vi "setMoveMode.vi"(0 "Controller in":refnum<class "_Controller.lvclass">, 2 "mode":T1, 5 "error in (no error)":errorcluster) -> (14 "Controller out":refnum<class "_Controller.lvclass">, 17 "success?":bool, 18 "response":string, 19 "error out":errorcluster)   [LabVIEW 2020, in "classes.lvlib" / "_Controller.lvclass"]
doc: "Sets the Move Mode to either ABSOLUTE or INCREMENTAL\n\nProduced By:\n\n<B>Kod Integrations, LLC</B>\n4835 Marianne Drive\nMount Airy, MD 21771\nhttp://www.kodintegrations.com\nemail: info@kodintegrations.com\nphone: (240) 687-1288"
uses:
  _Controller.lvclass
  common/controls/move_mode.ctl
  libraries/common.lvlib
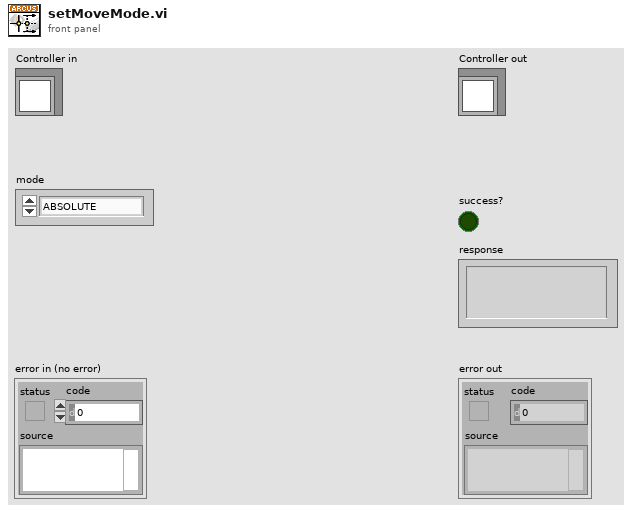
[diagram p1: front panel]
types:
  T1 = typedef "common.lvlib/move_mode.ctl" = enum16{"ABSOLUTE", "INCREMENTAL"}
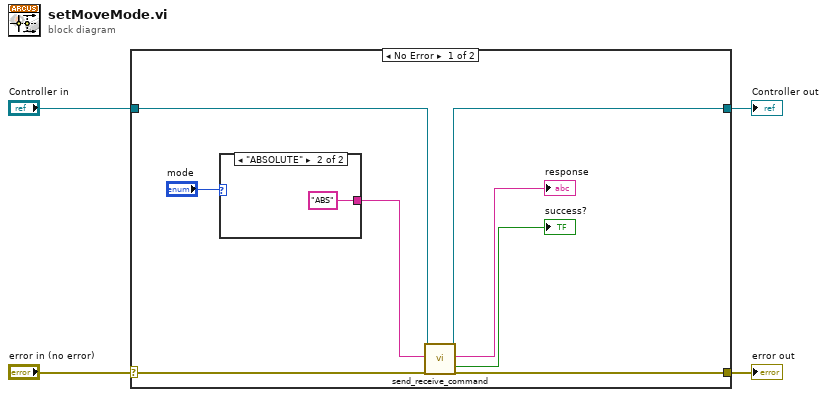
[diagram p0: block diagram]
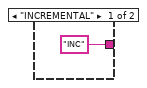
[diagram p2: hidden frame]
diagram:
  n1 = case shown="No Error" "error in (no error)" {
    selector: "error in (no error)" -> [w12 w16]
    tunnel: [w11 w16] -> w3
    tunnel: [w5 w15] -> w1
    tunnel: "Controller in" -> [w6 w15]
    frame No Error {
      n2 = case shown="\"ABSOLUTE\"" "mode" {
        tunnel: ["INC" "ABS"] -> w7
        frame "INCREMENTAL" {
        }
        frame "ABSOLUTE" {
        }
      }
      n3 = call "send_receive_command.vi"("reference (in)"=w6, "ASCII Command (in)"=w7, "error in (no error)"=w12) -> ("reference (out)"=w5:refnum<class "_Controller.lvclass">, "response (out)"=→"response":string, "success?"=→"success?":bool, "error out"=w11:errorcluster)  [unwired: 12 in, 1 out]
    }
    frame Error {
    }
  }
  "error out" <- w3
  "Controller out" <- w1
